vi "Write Read Visa Port Compare.vi"(7 "String in RX?":string, 8 "error in (no error)":errorcluster, 9 "Wait for read Msecs":dbl=500.0, 10 "write buffer":string, 11 "VISA Refnum in":refnum<visa-resource-name>) -> (0 "error out":errorcluster, 1 "In RX string?":bool, 2 "read buffer":string, 3 "VISA resource name out":refnum<visa-resource-name>)   [LabVIEW 2013]
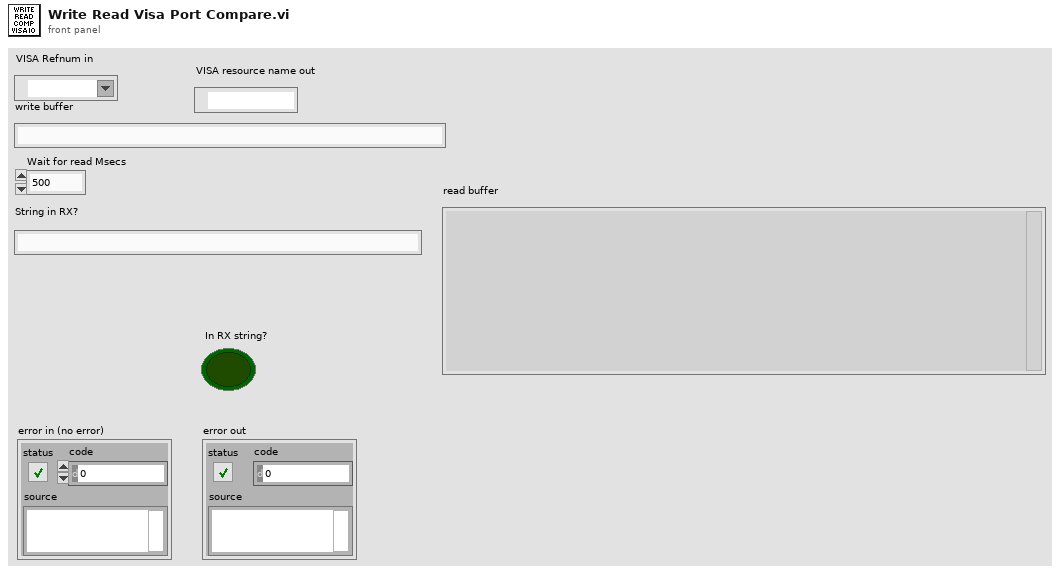
[diagram p1: front panel]
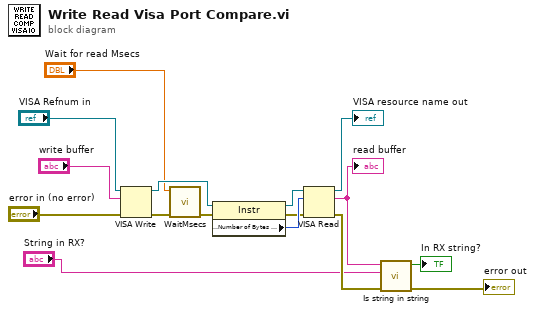
[diagram p0: block diagram]
diagram:
  n1 = VISA Write(VISA resource name="VISA Refnum in", write buffer="write buffer", error in (no error)="error in (no error)") -> (VISA resource name out=w13:refnum<visa-resource-name>, error out=w11:errorcluster)  [unwired: 1 out]
  n2 = call "WaitMsecs.vi"("error in (no error)"=w11, "Wait Msecs"="Wait for read Msecs") -> ("error out"=w12:errorcluster)  [unwired: 9 in]
  n3 = property class="Instr"(reference=w13, error in=w12) -> (reference out=w14:refnum<visa-resource-name>, error out=w15:errorcluster, "Serial Settings:Number of Bytes at Serial Port"=w16:u32)
  n4 = VISA Read(VISA resource name=w14, byte count=w16, error in (no error)=w15) -> (VISA resource name out=→"VISA resource name out":refnum<visa-resource-name>, read buffer=w4:string, error out=w5:errorcluster)  [unwired: 1 out]
  "read buffer" <- w4
  n5 = call "Is string in string.vi"("error in (no error)"=w5, "Search for string"="String in RX?", "String buffer"=w4) -> ("error out"=→"error out":errorcluster, "In string?"=→"In RX string?":bool)  [unwired: 7 in]
